vi "DSF.Engine.Plugin.Create.vi"(5 "Debug Flags":refnum<class "DSF.Engine.Debug Flags.lvclass">, 7 "transceiver count":i32, 8 "error in (no error)":errorcluster, 9 "Timing":refnum<class "DSF.Engine.Timing.lvclass">, 10 "Transceiver type":refnum<class "DSF.Engine.Transceiver.lvclass">, 11 "Transfer Groups":refnum<class "DSF.Engine.Transfer Group.lvclass">[](array[class])) -> (0 "error out":errorcluster, 2 "Transceiver":refnum<class "DSF.Engine.Transceiver.lvclass">, 3 "Plugin out":refnum<class "DSF.Engine.Plugin.lvclass">)   [LabVIEW 2017, in "DSF.Engine.lvlib" / "DSF.Engine.Plugin.lvclass"]
uses:
  DSF.Engine.Plugin.lvclass
  Timing/DSF.Engine.Timing.lvclass
  Transceiver/DSF.Engine.Transceiver.lvclass
  Transfer/DSF.Engine.Transfer Group.lvclass
  Debug/DSF.Engine.Debug Flags.lvclass
  DSF.Engine.Plugin.lvclass/DSF.Engine.Plugin.ctl
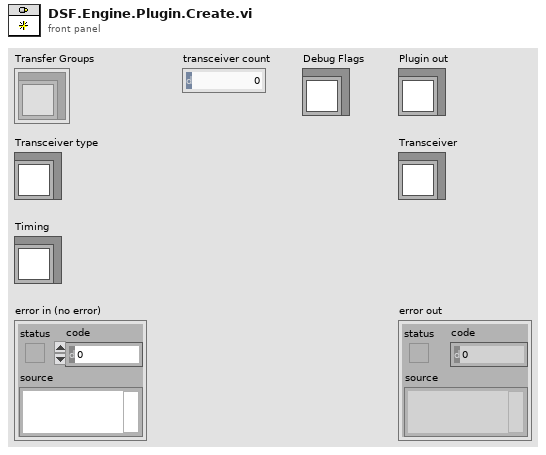
[diagram p1: front panel]
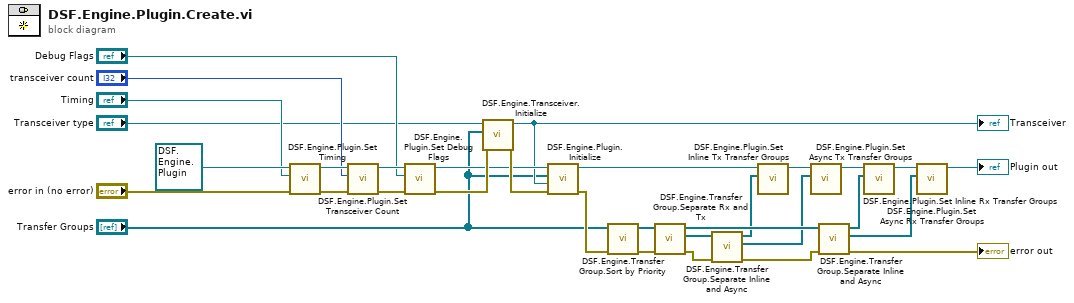
[diagram p0: block diagram]
diagram:
  n1 = call "DSF.Engine.Plugin.Set Timing.vi"("Timing"="Timing", "Plugin in"=refnum<class "DSF.Engine.Plugin.lvclass"> refnum) -> ("Plugin out"=w27:refnum<class "DSF.Engine.Plugin.lvclass">)  [unwired: 9 in]
  n2 = call "DSF.Engine.Plugin.Set Transceiver Count.vi"("transceiver count"="transceiver count", "Plugin in"=w27) -> ("Plugin out"=w14:refnum<class "DSF.Engine.Plugin.lvclass">)  [unwired: 9 in]
  n3 = call "DSF.Engine.Plugin.Set Debug Flags.vi"("Debug Flags"="Debug Flags", "Plugin in"=w14) -> ("Plugin out"=w3:refnum<class "DSF.Engine.Plugin.lvclass">)  [unwired: 9 in]
  n4 = call-dynamic "DSF.Engine.Transceiver.Initialize.vi"("error in (no error)"="error in (no error)", "Transfer Groups"="Transfer Groups", "Transceiver in"="Transceiver type") -> ("error out"=w4:errorcluster, "Transceiver out"=w2:refnum<class "DSF.Engine.Transceiver.lvclass">)  [unwired: 7 in]
  "Transceiver" <- w2
  n5 = call "DSF.Engine.Plugin.Initialize.vi"("error in (no error)"=w4, "Transceiver"=w2, "Transfer Groups"="Transfer Groups", "Plugin in"=w3) -> ("error out"=w10:errorcluster, "Plugin out"=w12:refnum<class "DSF.Engine.Plugin.lvclass">)  [unwired: 6 in]
  n6 = call "DSF.Engine.Transfer Group.Sort by Priority.vi"("error in (no error)"=w10, "Transfer Groups"="Transfer Groups") -> ("error out"=w29:errorcluster, "sorted Transfer Groups"=w28:refnum<class "DSF.Engine.Transfer Group.lvclass">[])  [unwired: 8 in]
  n7 = call "DSF.Engine.Transfer Group.Separate Rx and Tx.vi"("error in (no error)"=w29, "Transfer Groups"=w28) -> ("error out"=w25:errorcluster, "Tx Transfer Groups"=w24:refnum<class "DSF.Engine.Transfer Group.lvclass">[], "Rx Transfer Groups"=w23:refnum<class "DSF.Engine.Transfer Group.lvclass">[])  [unwired: 7 in]
  n8 = call "DSF.Engine.Transfer Group.Separate Inline and Async.vi"("error in (no error)"=w25, "Transfer Groups"=w24) -> ("error out"=w22:errorcluster, "Async Transfer Groups"=w20:refnum<class "DSF.Engine.Transfer Group.lvclass">[], "Inline Transfer Groups"=w21:refnum<class "DSF.Engine.Transfer Group.lvclass">[])  [unwired: 7 in]
  n9 = call "DSF.Engine.Plugin.Set Inline Tx Transfer Groups.vi"("Inline Tx Transfer Groups"=w21, "Plugin in"=w12) -> ("Plugin out"=w19:refnum<class "DSF.Engine.Plugin.lvclass">)  [unwired: 9 in]
  n10 = call "DSF.Engine.Plugin.Set Async Tx Transfer Groups.vi"("Async Tx Transfer Groups"=w20, "Plugin in"=w19) -> ("Plugin out"=w17:refnum<class "DSF.Engine.Plugin.lvclass">)  [unwired: 9 in]
  n11 = call "DSF.Engine.Transfer Group.Separate Inline and Async.vi"("error in (no error)"=w22, "Transfer Groups"=w23) -> ("error out"=→"error out":errorcluster, "Async Transfer Groups"=w15:refnum<class "DSF.Engine.Transfer Group.lvclass">[], "Inline Transfer Groups"=w18:refnum<class "DSF.Engine.Transfer Group.lvclass">[])  [unwired: 7 in]
  n12 = call "DSF.Engine.Plugin.Set Inline Rx Transfer Groups.vi"("Inline Rx Transfer Groups"=w18, "Plugin in"=w17) -> ("Plugin out"=w16:refnum<class "DSF.Engine.Plugin.lvclass">)  [unwired: 9 in]
  n13 = call "DSF.Engine.Plugin.Set Async Rx Transfer Groups.vi"("Async Rx Transfer Groups"=w15, "Plugin in"=w16) -> ("Plugin out"=→"Plugin out":refnum<class "DSF.Engine.Plugin.lvclass">)  [unwired: 9 in]
